vi "Init_Channels.vi"(11 "error in (no error)":errorcluster) -> (15 "error out":errorcluster)   [LabVIEW 2019, in "Service.lvlib"]
uses:
  Service.lvlib
  MsgQ/MsgQ.lvlib
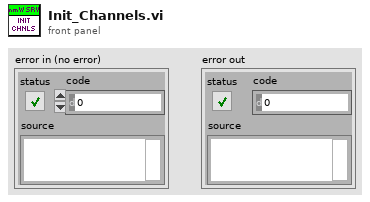
[diagram p1: front panel]
types:
  T1 = typedef "Service.lvlib/AppData.ctl" = cluster{"MsgQ":refnum<queue>, "Stop?":bool, "zmq sessions":cluster{"Control_endpoint":string, "Instr_endpoint":string}, "control-loop":cluster{"fromUI-Q":refnum<queue>, "toUI":refnum<user-event>, "Control_endpoint":string}, "UI-loop":cluster{"evnt_ref":refnum<event-registration>}, "logging":cluster{"level":dbl, "verbosity":dbl, "path":string, "Listener_ID":string}}
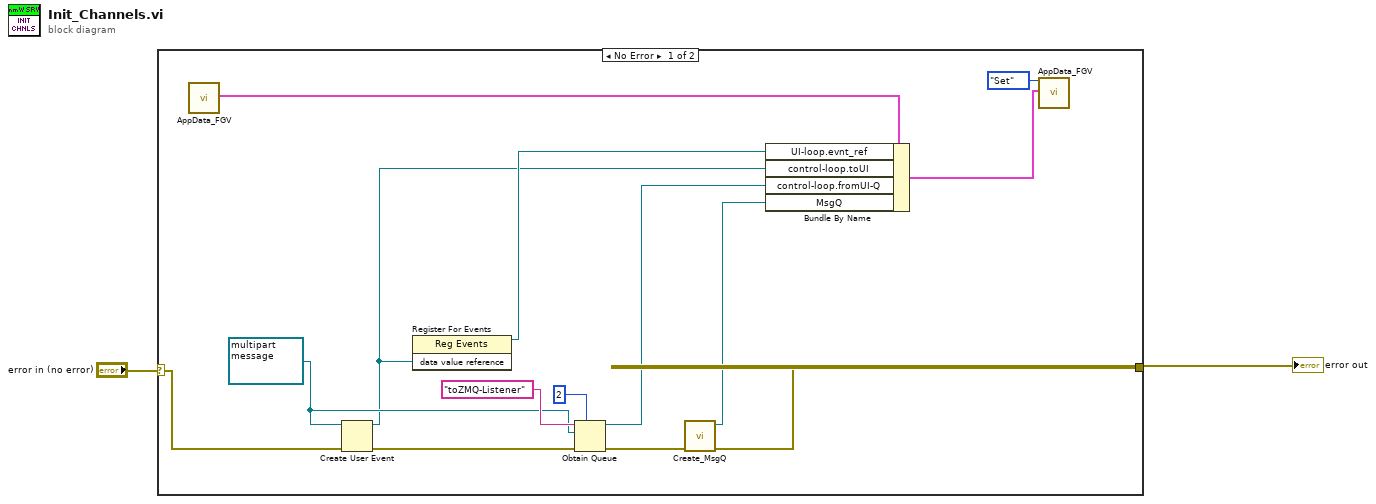
[diagram p0: block diagram]
diagram:
  n1 = case shown="No Error" "error in (no error)" {
    selector: "error in (no error)" -> [w4 w17]
    tunnel: [w5 w17] -> w2
    frame No Error {
      w14 = refnum<data-value> refnum ("data value reference")
      n2 = call "AppData_FGV.vi"() -> ("AppData out"=w13:T1)  [unwired: 18 in, 1 out]
      n3 = Create User Event(user event datatype=w14, error in=w4) -> (user event=w9:refnum<user-event>, error out=w3:errorcluster)
      n4 = register-events(w9) -> (reference out=w12:refnum<event-registration>)  [unwired: 2 in, 1 out]
      n5 = Obtain Queue(max queue size (-1, unlimited)=2, name (unnamed)="toZMQ-Listener", element data type=w14, error in (no error)=w3) -> (queue out=w8:refnum<queue>, error out=w7:errorcluster)  [unwired: 1 in, 1 out]
      n6 = call "Create_MsgQ.vi"("error in (no error)"=w7) -> ("error out"=w5:errorcluster, "Queue out"=w6:refnum<queue>)  [unwired: 9 in]
      n7 = Bundle By Name(cluster=w13, "UI-loop.evnt_ref"=w12, "control-loop.toUI"=w9, "control-loop.fromUI-Q"=w8, "MsgQ"=w6) -> (w11:T1)
      n8 = call "AppData_FGV.vi"("Mode"=enum16{"Get", "Set", "Reset"}."Set", "AppData in"=w11) -> ()  [unwired: 16 in, 2 out]
    }
    frame Error {
    }
  }
  "error out" <- w2
